vi "Cleanup.vi"(8 "error in (no error)":errorcluster, 11 "Windows System SAL in":refnum<class "Windows System SAL.lvclass">) -> (0 "error out":errorcluster)   [LabVIEW 2020, in "Volatus.lvlib" / "Windows System SAL.lvclass"]
uses:
  Windows System SAL.lvclass
  Windows System SAL.lvclass/Windows System SAL.ctl
  <vilib>/nisyscfg/nisyscfg.lvlib
  <vilib>/nisyscfg/Close (Hardware).vi
  <vilib>/nisyscfg/Close (System).vi
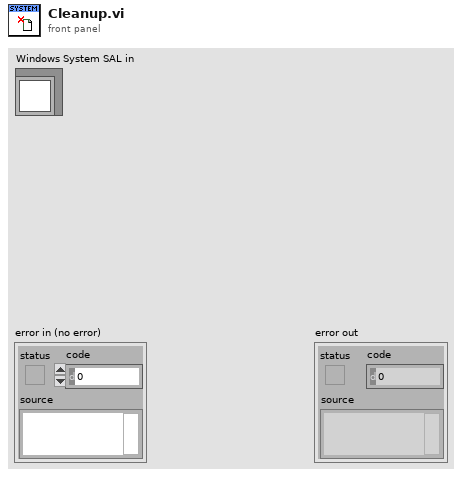
[diagram p1: front panel]
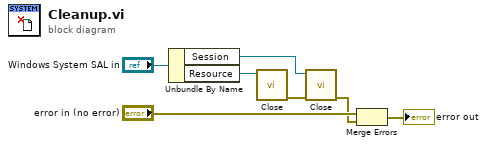
[diagram p0: block diagram]
diagram:
  n1 = Unbundle By Name("Windows System SAL in") -> ("Session"=w3:refnum<k21>, "Resource"=w4:refnum<k20>)
  n2 = call-poly <vilib>:"Close.vi"("Resource in"=w4) -> ("error out"=w5:errorcluster)  [unwired: 10 in]
  n3 = call-poly <vilib>:"Close.vi"("error in (no error)"=w5, "Session in"=w3) -> ("error out"=w1:errorcluster)  [unwired: 9 in]
  n4 = Merge Errors("error in (no error)", w1) -> (→"error out":errorcluster)
